vi "Configure Voltage Square Waveform.vi"(0 "VISA resource name":refnum<visa-resource-name>, 1 "Start Level (0 V)":dbl, 2 "Top Level (0 V)":dbl, 5 "Channel (1: Channel 1)":i32(ring)=1 items=["Channel 1"=1, "Channel 2"=2], 7 "Start Time (0.0001 s)":dbl=0.0001, 9 "End Time (0 s)":dbl, 11 "error in (no error)":errorcluster, 12 "Top Time (0.0001 s)":dbl=0.0001) -> (4 "VISA resource name out":refnum<visa-resource-name>, 15 "error out":errorcluster)   [LabVIEW 2012, in "Keysight B2980 Series.lvlib"]
doc: "Configures the voltage square waveform output.\n\n<b>Note(s):</b>\nThis VI is only applicable for model B2985A and B2987A."
uses:
  Keysight B2980 Series.lvlib
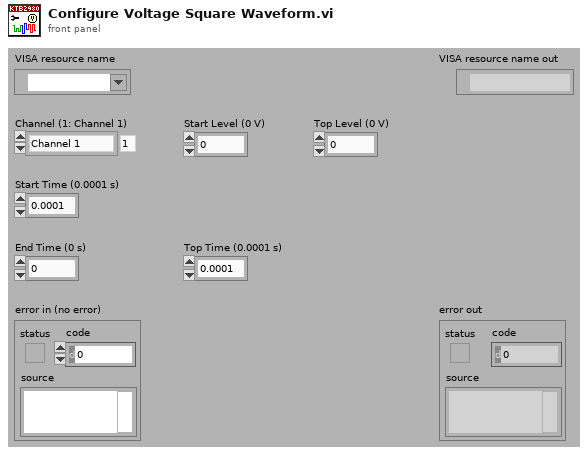
[diagram p1: front panel]
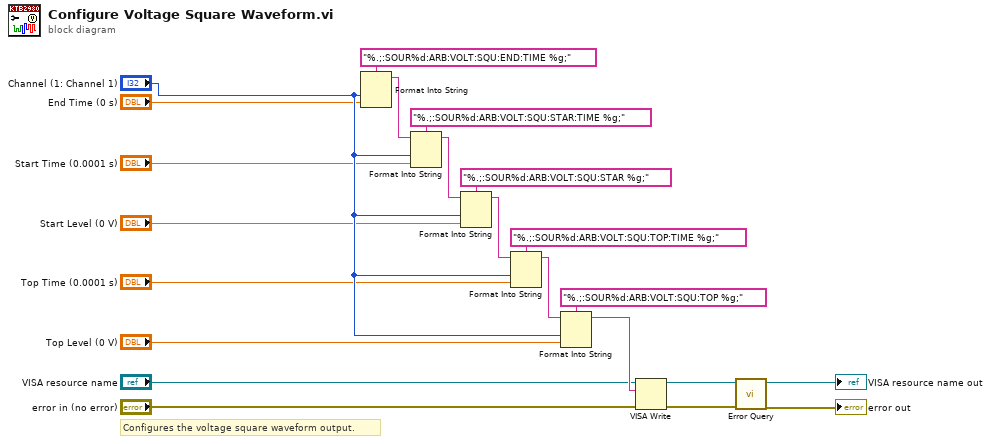
[diagram p0: block diagram]
diagram:
  # "Configures the voltage square waveform output."
  n1 = Format Into String(format string="%.;:SOUR%d:ARB:VOLT:SQU:END:TIME %g;", "Channel (1: Channel 1)", "End Time (0 s)") -> (resulting string=w19:string)  [unwired: 2 in, 1 out]
  n2 = Format Into String(format string="%.;:SOUR%d:ARB:VOLT:SQU:STAR:TIME %g;", initial string=w19, "Channel (1: Channel 1)", "Start Time (0.0001 s)") -> (resulting string=w1:string)  [unwired: 1 in, 1 out]
  n3 = Format Into String(format string="%.;:SOUR%d:ARB:VOLT:SQU:STAR %g;", initial string=w1, "Channel (1: Channel 1)", "Start Level (0 V)") -> (resulting string=w16:string)  [unwired: 1 in, 1 out]
  n4 = Format Into String(format string="%.;:SOUR%d:ARB:VOLT:SQU:TOP:TIME %g;", initial string=w16, "Channel (1: Channel 1)", "Top Time (0.0001 s)") -> (resulting string=w13:string)  [unwired: 1 in, 1 out]
  n5 = Format Into String(format string="%.;:SOUR%d:ARB:VOLT:SQU:TOP %g;", initial string=w13, "Channel (1: Channel 1)", "Top Level (0 V)") -> (resulting string=w10:string)  [unwired: 1 in, 1 out]
  n6 = VISA Write(VISA resource name="VISA resource name", write buffer=w10, error in (no error)="error in (no error)") -> (VISA resource name out=w7:refnum<visa-resource-name>, error out=w6:errorcluster)  [unwired: 1 out]
  n7 = call "Error Query.vi"("error in (no error)"=w6, "VISA resource name"=w7) -> ("error out"=→"error out":errorcluster, "VISA resource name out"=→"VISA resource name out":refnum<visa-resource-name>)  [unwired: 8 out]
